vi "EVT Camera Get U Int32Param Inc.vi"(9 "inc":u32, 10 "name":string, 11 "camera":u64) -> (1 "inc out":u32, 3 "function return":u32(ring))   [LabVIEW 2019, in "EmergentCameraC.lvlib"]
doc: "EMERGENTCAMERAC_API EVT_ERROR EVT_CameraGetUInt32ParamInc(Camera_Handle camera, const char* name, unsigned int* inc);"
uses:
  EmergentCameraC.lvlib
  emergentInstall_Windows/win64/eSDK/bin/EmergentCameraC.dll
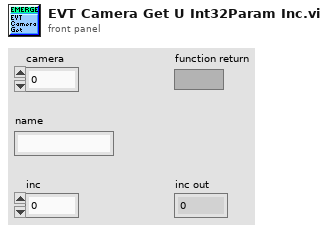
[diagram p1: front panel]
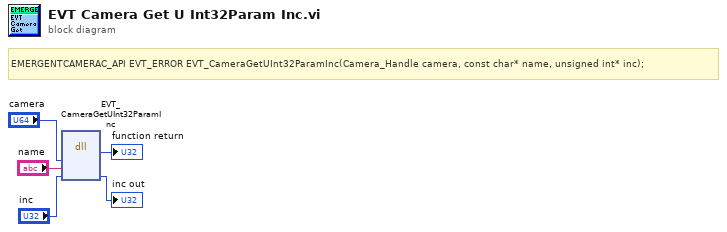
[diagram p0: block diagram]
diagram:
  # "EMERGENTCAMERAC_API EVT_ERROR EVT_CameraGetUInt32ParamInc(Camera_Handle camera, const char* name, unsigned int* inc);"
  n1 = dll-call lib="E:/emergent/host-new_QT/emergentInstall_Windows/win64/eSDK/bin/EmergentCameraC.*" fn="EVT_CameraGetUInt32ParamInc"("camera"="camera", "name"="name", "inc"="inc") -> (→"function return":u32, "inc"=→"inc out":u32)  [unwired: 5 in, 2 out]
